vi "JsonFormating.vi"   [LabVIEW 2019]
types:
  T1 = cluster{"id":u8, "checkIn":string, "checkOut":string, "work_hours":string, "employee":cluster{"id":u8, "name":string, "email":string, "uid":string, "hourly_rate":dbl, "hire_date":string, "job":cluster{"id":u8}, "createdAt":string}, "createdAt":string}
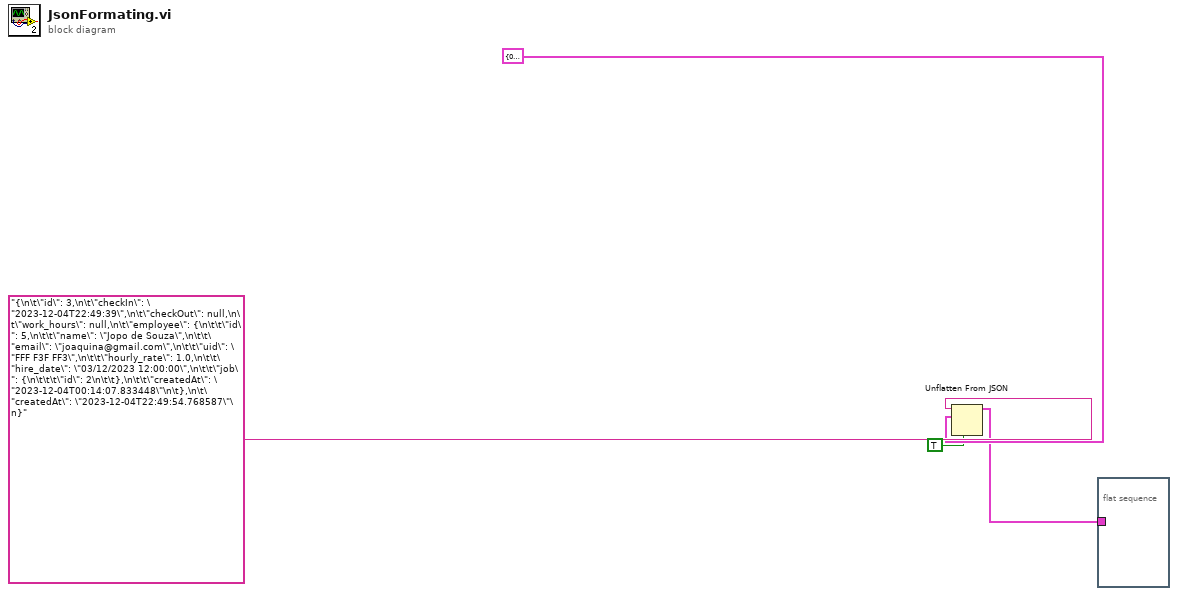
[diagram p0: block diagram]
diagram:
  n1 = Unflatten From JSON(JSON string="{\n\t\"id\": 3,\n\t\"checkIn\": \"2023-12-04T22:49:39\",\n\t\"checkOut\": null,\n\t\"work_hours\": null,\n\t\"employee\": {\n\t\t\"id\": 5,\n\t\t\"name\": \"Jopo de Souza\",\n\t\t\"email\": \"joaquina@gmail.com\",\n\t\t\"uid\": \"FFF F3F FF3\",\n\t\t\"hourly_rate\": 1.0,\n\t\t\"hire_date\": \"03/12/2023 12:00:00\",\n\t\t\"job\": {\n\t\t\t\"id\": 2\n\t\t},\n\t\t\"createdAt\": \"2023-12-04T00:14:07.833448\"\n\t},\n\t\"createdAt\": \"2023-12-04T22:49:54.768587\"\n}" ("Display"), type and defaults=T1 {"id"=0, "checkIn"="", "checkOut"="", "work_hours"="", "employee"={"id"=0, "name"="", "email"="", "uid"="", "hourly_rate"=0.0, "hire_date"="", "job"={"id"=0}, "createdAt"=""}, "createdAt"=""}, default null elements? (F)=TRUE) -> (value=w2:T1)  [unwired: 4 in, 1 out]
  n2 = flat-sequence {
    tunnel: w2 -> [_]
    frame #0 {
    }
  }
